vi "Run Bitfile.vi"() -> ()   [LabVIEW 2011]
uses:
  <vilib>/rvi/interface/nirviOpenFPGA/nirviOpenFPGA.xnode
  labview/FPGA Bitfiles/natcar_FPGATarget_Top-Level_610FB000.lvbitx
  <vilib>/FPGAPlugInAG/sbRIO-9606/niLvFpga_Open_sbRIO-9606.vi
  <vilib>/rvi/interface/common/dynamic/niFpgaDynamicAddResources.vi
  <vilib>/rvi/interface/nirviCloseFPGA/nirviCloseFPGA.xnode
  <vilib>/FPGAPlugInAG/Dynamic/niLvFpga_Close_Dynamic.vi
  <vilib>/Platform/TimedLoop/XDataNode/wakeup.ctl
  <vilib>/Platform/TimedLoop/XDataNode/XDNodeRunTimeDep.lvlib
  <vilib>/Platform/TimedLoop/XDataNode/nitl_modes.ctl
  <vilib>/Platform/TimedLoop/XDataNode/timing_clust.ctl
  <vilib>/Platform/TimedLoop/XDataNode/XDataNode.xnode
  <vilib>/rvi/interface/nirviReadWriteControl/nirviReadWriteControl.xnode
  NiFpgaLv.dll
  <vilib>/Utility/error.llb/Error Cluster From Error Code.vi
  <vilib>/rvi/interface/Simulation/niFpgaSimulationCallBeginRW.vi
  <vilib>/rvi/errors/niLvFpgaAdjustHostInterfaceError.vi
panel:
  out "Go Duty":u16
  out "Servo 1e-7s":u32
  out "Speed Error 2":dbl(graph)
  out "Line Error (cm)":dbl
  in  "Steering Kp":dbl min=0.0 max=1000.0 step=1.0
  out "really lost":bool
  out "line found":bool
  out "SC":bool
  out "S5":bool
  out "S4":bool
  out "S3":bool
  out "S2":bool
  out "S1":bool
  out "AI7":u16
  out "AI6":u16
  out "AI5":u16
  out "AI4":u16
  out "AI3":u16
  out "AI2":u16
  out "AI1":u16
  out "AI0":u16
  out "Speed Error":dbl(graph)
  in  "Offset":dbl=22.0 min=0.0 max=30.0 step=0.1
  out "Velocity counts":u32
  out "V [m/s]":dbl
  in  "RUN!":bool
  in  "Stop":bool
  in  "Kff":dbl=6.0 min=0.0 max=10.0 step=0.1
  in  "uBlaze Reset":bool
  in  "Steering ON 1e-7s":u32=15000 min=10240 max=19650 step=100
  in  "Steering":bool
  in  "Throttle":bool
  in  "GO frequency (Hz)":u16=1000 min=10 max=10000 step=10
  in  "GO duty (100*%)":u16 max=100 step=1
  in  "Vdes [m/s]":dbl min=0.0 max=5.0 step=0.1
  in  "Speed Ki":dbl=0.1 min=0.0 max=2.0 step=0.01
  in  "Throttle ON":bool
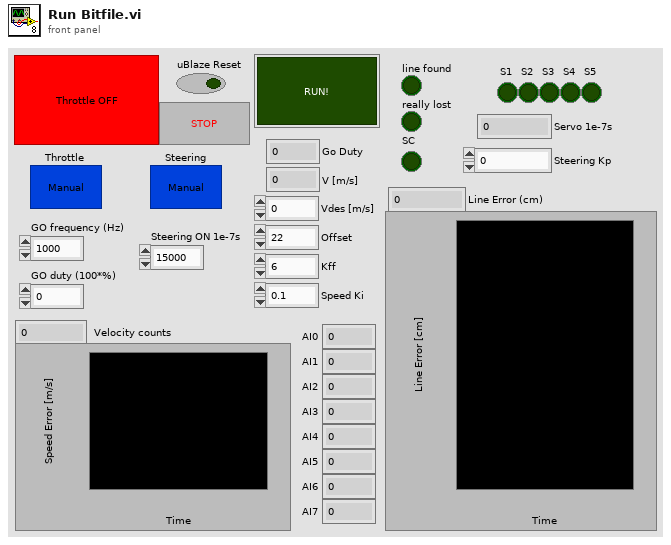
[diagram p1: front panel]
types:
  T1 = typedef "XDNodeRunTimeDep.lvlib/timing_clust.ctl" = cluster{"Expected End [f-1]":u64, "Actual End [f-1]":u64, "Finished Late? [f-1]":bool, "Expected End [i-1]":u64, "Actual End [i-1]":u64, "Finished Late? [i-1]":bool, "Expected Start [i]":u64, "Actual Start [i]":u64, "Expected Start [f]":u64, "Actual Start [f]":u64, "Source Name":string, "Structure Name":string, "Period":i64, "Deadline":i64, "Offset":i64, "Start":i64, "Priority":i32, "Timeout":i32, "Mode":T2, "Wakeup Reason":T3, "Error":errorcluster, "Source Type":string, "Secondary Source Type":string, "Global End Time":u64, "Global Start Time":u64, "Frame Duration":u64, "Iteration Duration":u64, "Assigned CPU":i32, "I/O Scan Engine Mode":u32}
  T2 = typedef "XDNodeRunTimeDep.lvlib/nitl_modes.ctl" = enum32{"No Change", "Process missed periods, maintain original phase", "Discard missed periods, maintain original phase", "Process missed periods, ignore original phase", "Discard missed periods, ignore original phase"}
  T3 = typedef "XDNodeRunTimeDep.lvlib/wakeup.ctl" = enum32{"Normal", "Aborted", "Asynchronous wakeup", "Timing source error", "Timed loop error", "Timeout"}
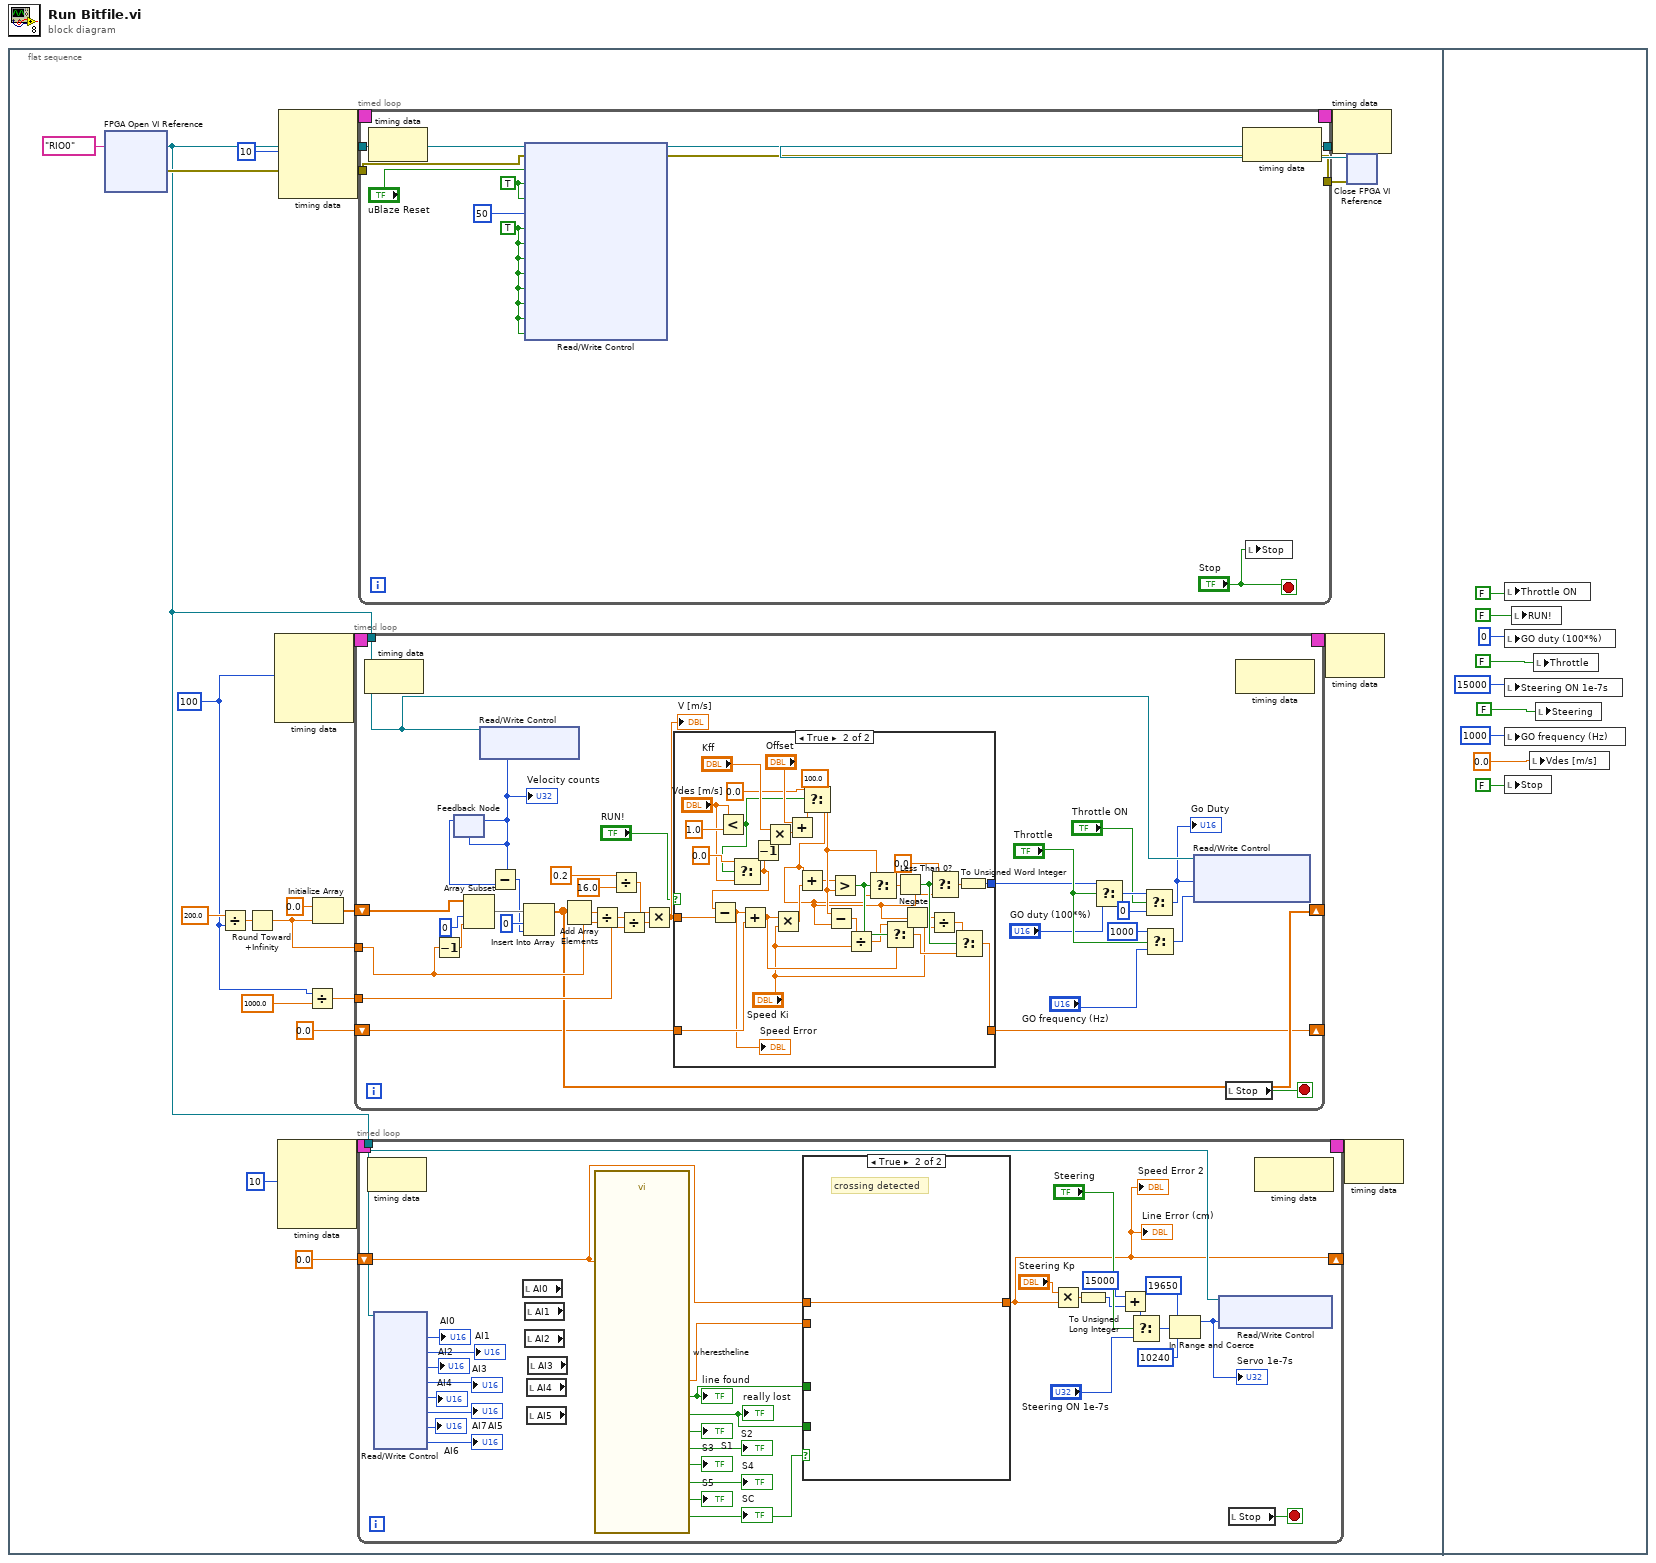
[diagram p0: block diagram]
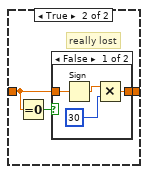
[diagram p4: hidden frame]
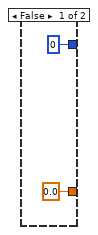
[diagram p6: hidden frame]
diagram:
  n1 = flat-sequence {
    frame #0 {
      w3 = i64 100 ("Period")
      n2 = xnode "FPGA Open VI Reference"("resource name"=tag "RIO0") -> ("FPGA VI Reference Out"=w2:refnum<k20>, "error out"=w16:errorcluster)  [unwired: 1 in]
      n3 = Divide(x=200.0, y=w3) -> (x/y=w10:dbl)
      n4 = Round Toward +Infinity(x=w10) -> (ceil(x): smallest int >= x=w9:dbl)
      n5 = node-c288(w3) -> (w23:T1)  [unwired: 3 in]
      n6 = node-c288(i64 10 ("Period")) -> (w21:T1)  [unwired: 3 in]
      n7 = node-c288(i64 10 ("Period")) -> (w19:T1)  [unwired: 3 in]
      n8 = Divide(x=w3, y=1000.0) -> (x/y=w5:dbl)
      n9 = Initialize Array(0.0 ("element"), w9) -> (w13:dbl[])
      n10 = timed-loop {
        timing: w23 -> [_]
        timing-out: [_] -> w22
        shift-right: [w126] -> _
        shift-left: w13 -> [w125]
        tunnel: w9 -> [w128]
        tunnel: w5 -> [w127]
        shift-right: [w123] -> _
        shift-left: 0.0 -> [w124]
        tunnel: w2 -> [w122]
        stop <- w121 stop-if-true
        n11 = node-c288() -> ()  [unwired: 1 in, 1 out]
        n12 = Decrement(x=w128) -> (x-1=w109:dbl)
        n13 = Array Subset(array=w125, index=0, length=w109) -> (w101:dbl[])
        n14 = xnode "Read/Write Control"("FPGA VI Reference In"=w122) -> ("Velocity counts"=w97:u32)  [unwired: 1 in, 2 out]
        "Velocity counts" <- w97
        n15 = feedback #1(w97) -> (w98:u32)
        n16 = feedback-in #1(w97) -> ()
        n17 = Subtract(x=w97, y=w98) -> (x-y=w100:u32)
        n18 = Insert Into Array(array=w101, index=0, new element=w100) -> (w126:dbl[])
        n19 = Add Array Elements(numeric array=w126) -> (sum=w99:dbl)
        n20 = Divide(x=w99, y=w128) -> (x/y=w107:dbl)
        n21 = Divide(x=0.2, y=16.0) -> (x/y=w103:dbl)
        n22 = Divide(x=w107, y=w127) -> (x/y=w104:dbl)
        n23 = Multiply(x=w103, y=w104) -> (x*y=w102:dbl)
        "V [m/s]" <- w102
        n24 = case shown="True" "RUN!" {
          tunnel: w124 -> [_ w162]
          tunnel: [0.0 w161] -> w123
          tunnel: [u16 0 w160] -> w116
          tunnel: w102 -> [_ w159]
          frame False {
          }
          frame True {
            w153 = 100.0 ("y")
            n25 = Less?(x="Vdes [m/s]", y=1.0) -> (x < y?=w135:bool)
            n26 = Select(t=0.0, s=w135, f="Vdes [m/s]") -> (s? t:f=w136:dbl)
            n27 = Subtract(x=w136, y=w159) -> (x-y=w131:dbl)
            "Speed Error" <- w131
            n28 = Add(x=w131, y=w162) -> (x+y=w146:dbl)
            n29 = Decrement(x=w136) -> (x-1=w137:dbl)
            n30 = Multiply(x="Kff", y=w137) -> (x*y=w140:dbl)
            n31 = Multiply(x=w146, y="Speed Ki") -> (x*y=w158:dbl)
            n32 = Add(x="Offset", y=w140) -> (x+y=w133:dbl)
            n33 = Select(t=0.0, s=w135, f=w133) -> (s? t:f=w132:dbl)
            n34 = Add(x=w132, y=w158) -> (x+y=w149:dbl)
            n35 = Subtract(x=w153, y=w132) -> (x-y=w152:dbl)
            n36 = Greater?(x=w149, y=w153) -> (0:w154:bool)
            n37 = Divide(x=w152, y="Speed Ki") -> (x/y=w151:dbl)
            n38 = Select(t=w153, s=w154, f=w132) -> (s? t:f=w155:dbl)
            n39 = Select(t=w151, s=w154, f=w146) -> (s? t:f=w144:dbl)
            n40 = Less Than 0?(x=w155) -> (x < 0?=w150:bool)
            n41 = Negate(x=w132) -> (-x=w148:dbl)
            n42 = Divide(x=w148, y="Speed Ki") -> (x/y=w147:dbl)
            n43 = Select(t=0.0, s=w150, f=w132) -> (s? t:f=w145:dbl)
            n44 = Select(t=w147, s=w150, f=w144) -> (s? t:f=w161:dbl)
            n45 = To Unsigned Word Integer(number=w145) -> (unsigned 16bit integer=w160:u16)
          }
        }
        n46 = Select(t=w116, s="Throttle", f="GO duty (100*%)") -> (s? t:f=w113:u16)
        n47 = Select(t=w113, s="Throttle ON", f=u16 0 ("t")) -> (s? t:f=w112:u16)
        "Go Duty" <- w112
        n48 = Select(t=u16 1000, s="Throttle", f="GO frequency (Hz)") -> (s? t:f=w115:u16)
        n49 = xnode "Read/Write Control"("FPGA VI Reference In"=w122, "GO duty (100*%)"=w112, "GO frequency (Hz)"=w115) -> ()  [unwired: 1 in, 2 out]
        n50 = local read "Stop"() -> (w121:bool)
        n51 = node-c288() -> ()  [unwired: 1 in, 1 out]
      }
      n52 = timed-loop {
        timing: w21 -> [_]
        timing-out: [_] -> w20
        tunnel: w2 -> [w40]
        shift-right: [w39] -> _
        shift-left: 0.0 -> [w54]
        stop <- w69 stop-if-true
        n53 = node-c288() -> ()  [unwired: 1 in, 1 out]
        n54 = xnode "Read/Write Control"("FPGA VI Reference In"=w40) -> ("AI0"=→"AI0":u16, "AI1"=→"AI1":u16, "AI2"=→"AI2":u16, "AI3"=→"AI3":u16, "AI4"=→"AI4":u16, "AI5"=→"AI5":u16, "AI6"=→"AI6":u16, "AI7"=→"AI7":u16)  [unwired: 1 in, 2 out]
        n55 = local read "AI0"() -> ()  [unwired: 1 out]
        n56 = local read "AI1"() -> ()  [unwired: 1 out]
        n57 = local read "AI2"() -> ()  [unwired: 1 out]
        n58 = local read "AI4"() -> ()  [unwired: 1 out]
        n59 = local read "AI5"() -> ()  [unwired: 1 out]
        n60 = local read "AI3"() -> ()  [unwired: 1 out]
        n61 = call "wherestheline.vi"("last error"=w54) -> ("SC"=w50:bool, "error"=w53:dbl, "line found"=w55:bool, "really lost"=w51:bool, "S1"=→"S1":bool, "S2"=→"S2":bool, "S3"=→"S3":bool, "S4"=→"S4":bool, "S5"=→"S5":bool)  [unwired: 18 in]
        "SC" <- w50
        "line found" <- w55
        "really lost" <- w51
        n62 = case shown="True" w50 {
          tunnel: w55 -> [w75 _]
          tunnel: w54 -> [w74 w89]
          tunnel: w53 -> [w73 _]
          tunnel: [w72 w89] -> w39
          tunnel: w51 -> [w71 _]
          frame False {
            # "no crossing"
            n63 = case shown="True" w75 {
              tunnel: w74 -> [w77 _]
              tunnel: w73 -> [_ w88]
              tunnel: [w76 w88] -> w72
              tunnel: w71 -> [w78 _]
              frame False {
                # "line not found"
                n64 = case shown="False" w78 {
                  tunnel: [w79 w81] -> w76
                  tunnel: w77 -> [w79 w80]
                  frame False {
                    # "not really lost"
                  }
                  frame True {
                    # "really lost"
                    n65 = Equal To 0?(x=w80) -> (x = 0?=w82:bool)
                    n66 = case shown="False" w82 {
                      tunnel: [w83 w87] -> w81
                      tunnel: w80 -> [w86 w87]
                      frame False {
                        n67 = Sign(1:w86) -> (0:w85:dbl)
                        n68 = Multiply(x=w85, y=u16 30) -> (x*y=w83:dbl)
                      }
                      frame True {
                      }
                    }
                  }
                }
              }
              frame True {
                # "line is found"
              }
            }
          }
          frame True {
            # "crossing detected"
          }
        }
        "Line Error (cm)" <- w39
        "Speed Error 2" <- w39
        n69 = Multiply(x="Steering Kp", y=w39) -> (x*y=w48:dbl)
        n70 = To Unsigned Long Integer(number=w48) -> (unsigned 32bit integer=w46:u32)
        n71 = Add(x=u32 15000, y=w46) -> (x+y=w47:u32)
        n72 = Select(t=w47, s="Steering", f="Steering ON 1e-7s") -> (s? t:f=w44:u32)
        n73 = In Range and Coerce(upper limit=u32 19650, x=w44, lower limit=u32 10240) -> (coerced(x)=w41:u32)  [unwired: 1 out]
        "Servo 1e-7s" <- w41
        n74 = xnode "Read/Write Control"("FPGA VI Reference In"=w40, "Steering ON 1e-7s"=w41) -> ()  [unwired: 1 in, 2 out]
        n75 = local read "Stop"() -> (w69:bool)
        n76 = node-c288() -> ()  [unwired: 1 in, 1 out]
      }
      n77 = timed-loop {
        tunnel: w2 -> [w32]
        tunnel: [w31] -> w17
        tunnel: w16 -> [w29]
        tunnel: [w28] -> w15
        timing: w19 -> [_]
        timing-out: [_] -> w18
        stop <- "Stop" stop-if-true
        w24 = TRUE ("Enable AI0")
        w27 = TRUE ("manual steering")
        n78 = node-c288() -> ()  [unwired: 1 in, 1 out]
        n79 = xnode "Read/Write Control"("FPGA VI Reference In"=w32, "error in"=w29, "uBlaze Reset"="uBlaze Reset", "manual steering"=w27, "manual throttle"=w27, "Steering frequency (Hz)"=u16 50, "Enable AI0"=w24, "Enable AI1"=w24, "Enable AI2"=w24, "Enable AI3"=w24, "Enable AI4"=w24, "Enable AI5"=w24, "Enable AI6"=w24, "Enable AI7"=w24) -> ("FPGA VI Reference Out"=w31:refnum<k20>, "error out"=w28:errorcluster)
        n80 = node-c288() -> ()  [unwired: 1 in, 1 out]
        n81 = local write "Stop"("Stop") -> ()
      }
      n82 = node-c288(w22) -> ()  [unwired: 1 out]
      n83 = node-c288(w18) -> ()  [unwired: 1 out]
      n84 = node-c288(w20) -> ()  [unwired: 1 out]
      n85 = xnode "Close FPGA VI Reference"("FPGA VI Reference In"=w17, "error in"=w15) -> ()  [unwired: 1 out]
    }
    frame #1 {
      n86 = local write "Throttle ON"(FALSE ("Throttle ON")) -> ()
      n87 = local write "GO duty (100*%)"(u16 0 ("GO duty (100*%)")) -> ()
      n88 = local write "Steering ON 1e-7s"(u32 15000 ("Steering ON 1e-7s")) -> ()
      n89 = local write "GO frequency (Hz)"(u16 1000 ("GO frequency (Hz)")) -> ()
      n90 = local write "Stop"(FALSE ("Stop")) -> ()
      n91 = local write "RUN!"(FALSE ("START!")) -> ()
      n92 = local write "Vdes [m/s]"(0.0 ("Desired Speed [m/s]")) -> ()
      n93 = local write "Throttle"(FALSE ("Automatic Throttle")) -> ()
      n94 = local write "Steering"(FALSE ("Automatic Steering")) -> ()
    }
  }
